vi "move_when_dist_less_dhan_10.vi"() -> ()   [LabVIEW 2014, in "poiuy.lvrbt"]
uses:
  poiuy.lvrbt
  <vilib>/NXT/Dual Mode Library/Sensors/EV3_Ultrasonic_CM.vi
  <vilib>/NXT/LegoClasses/BrickReference/BrickReference.lvclass
  <vilib>/NXT/Subs/LVHSConnector.ctl
  <vilib>/NXT/NXTIO Xnodes/NXTIOXNode/NXTIO.xnode
  <vilib>/NXT/NXTIO Xnodes/AddressXNode/NXTIOAddress.xnode
  <vilib>/NXT/Block Support/NXT_OutputPort.ctl
  <vilib>/NXT/NXTIO Xnodes/NXTIONodeSubVIs/NXTMoveMotors.vi
  <vilib>/NXT/NXTIO Xnodes/NXTIONodeSubVIs/NXTStopMotors.vi
panel:
  in  "stop":bool
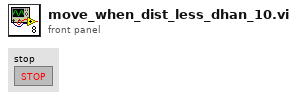
[diagram p1: front panel]
types:
  T1 = typedef "NXT_OutputPort.ctl" = u8
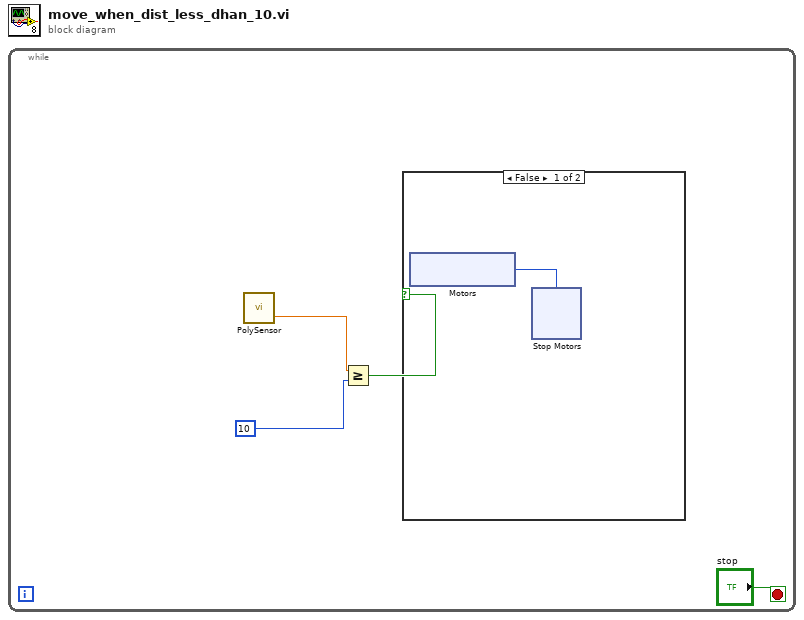
[diagram p0: block diagram]
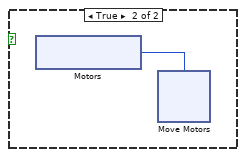
[diagram p2: hidden frame]
diagram:
  n1 = while {
    stop <- "stop" stop-if-true
    n2 = call-poly <vilib>:"PolySensor.vi"() -> ("Centimeters"=w4:sgl)  [unwired: 3 in, 1 out]
    n3 = Greater Or Equal?(x=w4, y=10) -> (x >= y?=w2:bool)
    n4 = case shown="False" w2 {
      frame False {
        n5 = xnode "Motors"() -> ("Motor"=w5:T1)
        n6 = xnode "Stop Motors"("Motors"=w5) -> ()  [unwired: 1 in, 1 out]
      }
      frame True {
        n7 = xnode "Motors"() -> ("Motor"=w12:T1)
        n8 = xnode "Move Motors"("Motors"=w12) -> ()  [unwired: 2 in, 1 out]
      }
    }
  }
